vi "timer api.vi"(11 "Boolean 3":bool) -> (3 "x .and. y? 2":bool)   [LabVIEW 2015]
panel:
  in  "Boolean 2":bool
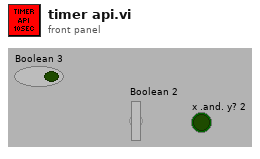
[diagram p1: front panel]
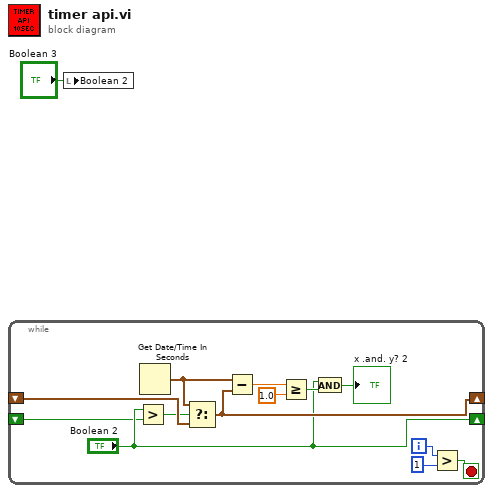
[diagram p0: block diagram]
diagram:
  n1 = while {
    shift-right: [w11] -> _
    shift-left: _ -> [w14]
    shift-right: ["Boolean 2"] -> _
    shift-left: _ -> [w5]
    i -> [w4]
    stop <- w2 stop-if-true
    n2 = Greater?(x="Boolean 2", y=w5) -> (0:w13:bool)
    n3 = Get Date/Time In Seconds() -> (seconds since 1Jan1904=w12:timestamp)
    n4 = Select(t=w12, s=w13, f=w14) -> (s? t:f=w11:timestamp)
    n5 = Subtract(x=w12, y=w11) -> (x-y=w10:dbl)
    n6 = Greater Or Equal?(x=w10, y=1.0) -> (x >= y?=w8:bool)
    n7 = And(x="Boolean 2", y=w8) -> (x .and. y?=→"x .and. y? 2":bool)
    n8 = Greater?(x=w4, y=1) -> (0:w2:bool)
  }
  n9 = local write "Boolean 2"("Boolean 3") -> ()
